vi "SerialArray.vi"(0 "COMPORT":refnum<visa-resource-name>="COM4", 5 "Delay Time (ms)":dbl=1.0 caption="Delay Time (s)", 11 "error in (no error)":errorcluster, 12 "Command ( ; seperation)":string, 13 "Open Serial":bool, 14 "Close Serial":bool) -> (1 "time(s)":dbl=0.17611279999982798, 2 "Success":bool[](array[boolean]), 3 "All Success":bool, 4 "comport":refnum<visa-resource-name>="COM4", 6 "Array":string[](array[string]), 8 "string":string="caladc\r\n>\ncaladc -r\r\ncaladc delay: 0x00004333\r\n>\r\n", 15 "error out":errorcluster)   [LabVIEW 2018]
panel:
  out "output 2":string
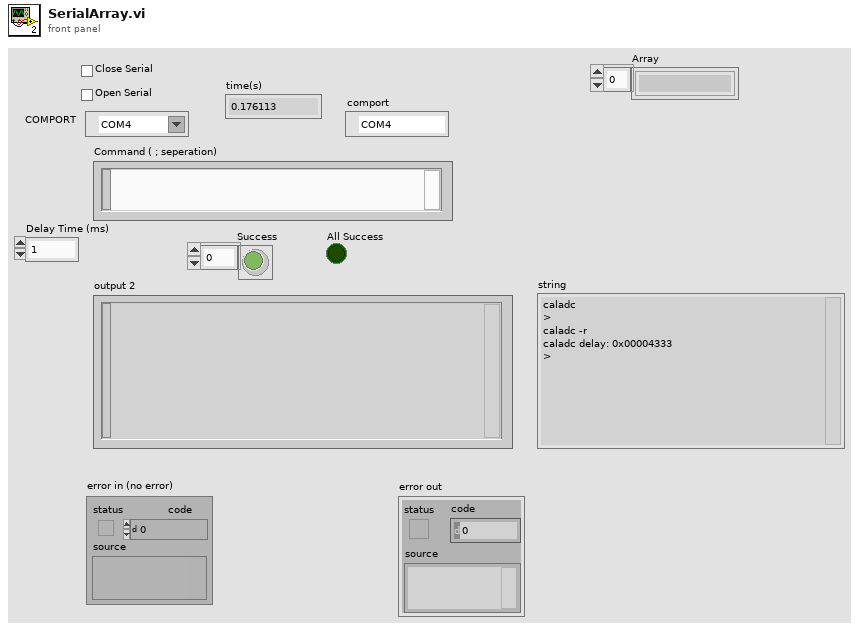
[diagram p1: front panel]
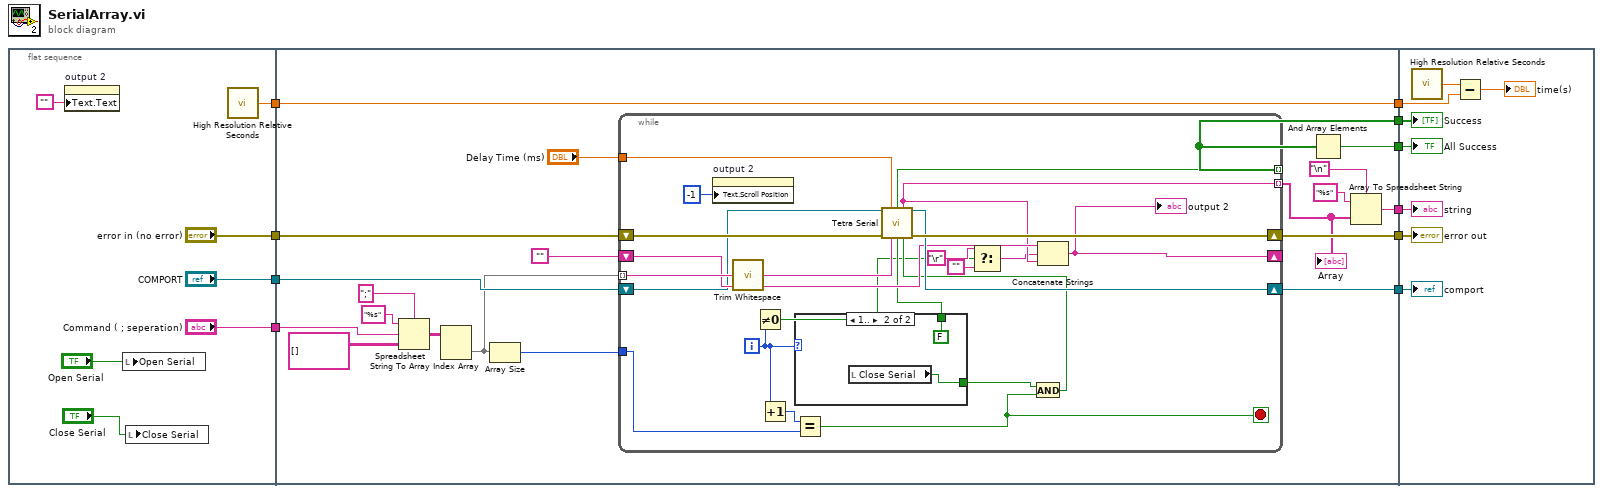
[diagram p0: block diagram]
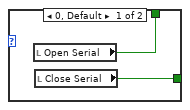
[diagram p2: hidden frame]
diagram:
  n1 = flat-sequence {
    tunnel: ["error in (no error)"] -> w5
    tunnel: ["COMPORT"] -> w4
    tunnel: ["Command ( ; seperation)"] -> w3
    tunnel: [w14] -> w2
    tunnel: [w33] -> w10
    tunnel: [w30] -> w9
    tunnel: [w28] -> w8
    tunnel: [w23] -> w7
    tunnel: [w20] -> w6
    tunnel: w5 -> [w32]
    tunnel: w4 -> [w31]
    tunnel: w3 -> [w25]
    tunnel: w2 -> [w19]
    tunnel: [w19] -> w1
    tunnel: w10 -> [w69]
    tunnel: w9 -> [w70]
    tunnel: w8 -> [w71]
    tunnel: w7 -> [w72]
    tunnel: w6 -> [w68]
    tunnel: w1 -> [w66]
    frame #0 {
      n2 = property on="output 2" class="Str"("Text.Text"="") -> ()  [unwired: 2 in, 2 out]
      n3 = local write "Open Serial"("Open Serial") -> ()
      n4 = local write "Close Serial"("Close Serial") -> ()
      n5 = call <vilib>:"High Resolution Relative Seconds.vi"() -> ("relative seconds"=w14:dbl)
    }
    frame #1 {
      n6 = Spreadsheet String To Array(delimiter (Tab)=";", format string="%s", spreadsheet string=w25, array type (2D Dbl)=string[][] []) -> (array=w34:string[][])
      n7 = Index Array(array=w34) -> (element=w29:string[])  [unwired: 2 in]
      n8 = Array Size(array=w29) -> (size(s)=w21:i32)
      n9 = while {
        shift-right: [w60] -> w33
        shift-left: w32 -> [w59]
        shift-right: [w58] -> w30
        shift-left: w31 -> [w50]
        tunnel: [w54] -> w22 mode=indexing
        tunnel: w29 -> [w57] mode=indexing
        tunnel: w21 -> [w47]
        shift-right: [w51] -> _
        shift-left: "" -> [w55]
        tunnel: [w52] -> w20 mode=indexing
        tunnel: "Delay Time (ms)" -> [w43]
        i -> [w39]
        stop <- w46 stop-if-true
        n10 = property on="output 2" class="Str"("Text.Scroll Position"=-1) -> ()  [unwired: 2 in, 2 out]
        n11 = call <vilib>:"Trim Whitespace.vi"("string"=w57) -> ("trimmed string"=w53:string)  [unwired: 1 in]
        n12 = Not Equal To 0?(x=w39) -> (x != 0?=w40:bool)
        n13 = Increment(x=w39) -> (x+1=w48:i32)
        n14 = case shown="1.." w39 {
          tunnel: [w62 FALSE ("Open Serial")] -> w49
          tunnel: [w61 w63] -> w45
          frame 0, Default {
            n15 = local read "Open Serial"() -> (w62:bool)
            n16 = local read "Close Serial"() -> (w61:bool)
          }
          frame 1.. {
            n17 = local read "Close Serial"() -> (w63:bool)
          }
        }
        n18 = Equal?(x=w48, y=w47) -> (x = y?=w46:bool)
        n19 = Select(t="\r", s=w40, f="") -> (s? t:f=w42:string)
        n20 = And(x=w45, y=w46) -> (x .and. y?=w44:bool)
        n21 = call "Tetra Serial.vi"("COMPORT"=w50, "Delay Time (ms)"=w43, "error in (no error)"=w59, "Command"=w53, "Open Ser(t)"=w49, "Close Ser(t)"=w44) -> ("Success"=w52:bool, "output"=w54:string, "comport"=w58:refnum<visa-resource-name>, "error out"=w60:errorcluster)  [unwired: 6 in]
        n22 = Concatenate Strings(w55, w42, w54) -> (w51:string)
        "output 2" <- w51
      }
      "Array" <- w22
      n23 = And Array Elements(Boolean array=w20) -> (logical AND=w23:bool)
      n24 = Array To Spreadsheet String(delimiter (Tab)="\n", array=w22, 3:"%s" ("format string")) -> (spreadsheet string=w28:string)
    }
    frame #2 {
      n25 = call <vilib>:"High Resolution Relative Seconds.vi"() -> ("relative seconds"=w67:dbl)
      n26 = Subtract(x=w67, y=w66) -> (x-y=→"time(s)":dbl)
      "error out" <- w69
      "comport" <- w70
      "Success" <- w68
      "string" <- w71
      "All Success" <- w72
    }
  }
